vi "Set Channel DC Offset.vi"(8 "error in (no error)":errorcluster, 10 "Params":variant, 11 "PI650 VoltageAmp in":refnum<class "PI650 VoltageAmp.lvclass">) -> (0 "error out":errorcluster, 3 "PI650 VoltageAmp out":refnum<class "PI650 VoltageAmp.lvclass">)   [LabVIEW 2020, in "Pickering.lvlib" / "PI650 VoltageAmp.lvclass"]
uses:
  PI650 VoltageAmp.lvclass
  TypeDefs/Channel DC offset.ctl
  PI650 VoltageAmp.lvclass/PI650 VoltageAmp.ctl
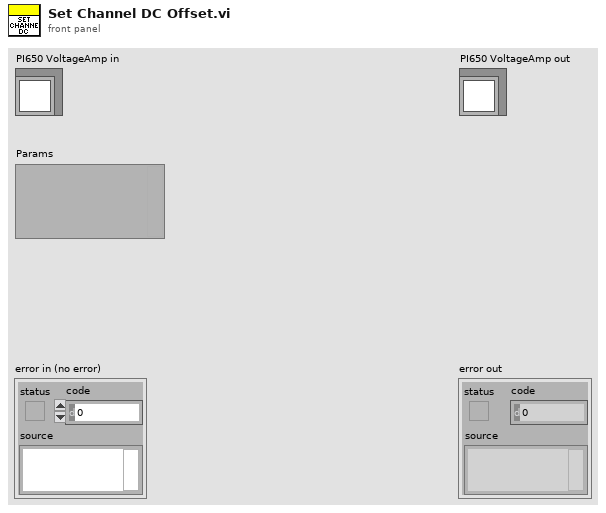
[diagram p1: front panel]
types:
  T1 = typedef "Pickering.lvlib/PI650 VoltageAmp.lvclass/Channel DC offset.ctl" = cluster{"Channel (CH1)":u32, "Offset (128)":u32}
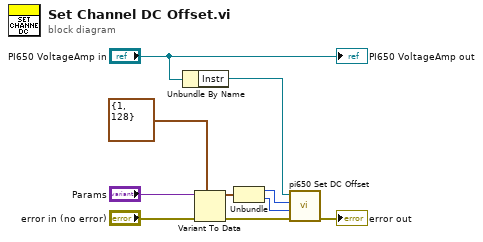
[diagram p0: block diagram]
diagram:
  n1 = Unbundle By Name("PI650 VoltageAmp in") -> ("Instr"=w9:refnum<visa-resource-name>)
  n2 = Variant To Data(error in="error in (no error)", type=T1 {"Channel (CH1)"=1, "Offset (128)"=128}, Variant="Params") -> (data=w3:T1, error out=w5:errorcluster)
  n3 = Unbundle(w3) -> ("Channel (CH1)"=w2:u32, "Offset (128)"=w1:u32)
  n4 = call <instrlib>:"pi650 Set DC Offset.vi"("error in (no error)"=w5, "Offset (128)"=w1, "Channel (0)"=w2, "instrument handle"=w9) -> ("error out"=→"error out":errorcluster)  [unwired: 6 in, 1 out]
  "PI650 VoltageAmp out" <- "PI650 VoltageAmp in"
